vi "Get_Joystick.vi"(1 "Joystick_One":string="Pilot Controller", 2 "Joystick_Two":string="CoPilot Controller") -> (6 "Joystick_Out":T1)   [LabVIEW 2020]
uses:
  Joystick_Controls.ctl
  <vilib>/Rock Robotics/WPI/Joystick/WPI_JoystickDeviceEnum.ctl
  <vilib>/Rock Robotics/WPI/Utilities/WPI_GetSetVariantRefNum.vi
panel:
  in  "Joystick Controls":T1
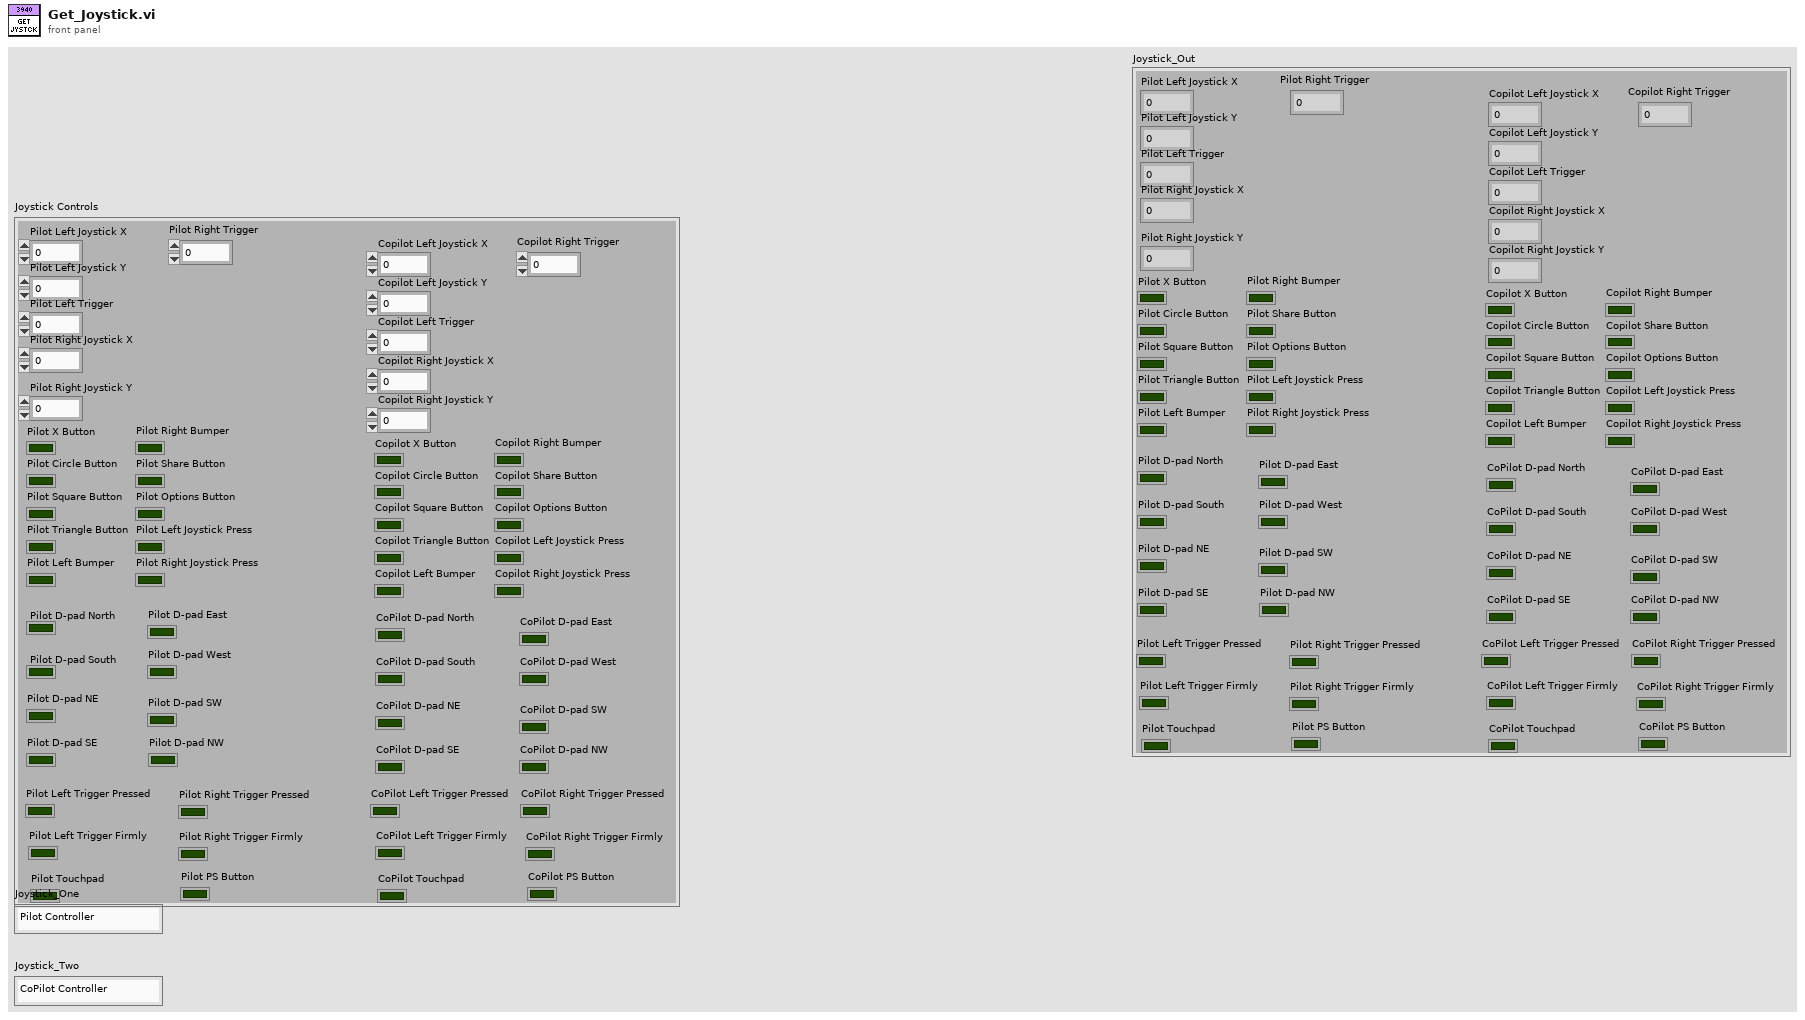
[diagram p1: front panel]
types:
  T1 = typedef "Joystick_Controls.ctl" = cluster{"Pilot Left Joystick X":dbl, "Pilot Left Joystick Y":dbl, "Pilot X Button":bool, "Pilot Circle Button":bool, "Pilot Square Button":bool, "Pilot Triangle Button":bool, "Pilot Left Bumper":bool, "Pilot Right Bumper":bool, "Pilot Share Button":bool, "Pilot Options Button":bool, "Pilot Left Joystick Press":bool, "Pilot Right Joystick Press":bool, "Pilot Left Trigger":dbl, "Pilot Right Joystick X":dbl, "Pilot Right Joystick Y":dbl, "Pilot Right Trigger":dbl, "Copilot Left Joystick X":dbl, "Copilot Left Joystick Y":dbl, "Copilot X Button":bool, "Copilot Circle Button":bool, "Copilot Square Button":bool, "Copilot Triangle Button":bool, "Copilot Left Bumper":bool, "Copilot Right Bumper":bool, "Copilot Share Button":bool, "Copilot Options Button":bool, "Copilot Left Joystick Press":bool, "Copilot Right Joystick Press":bool, "Copilot Left Trigger":dbl, "Copilot Right Joystick X":dbl, "Copilot Right Joystick Y":dbl, "Copilot Right Trigger":dbl, "Pilot D-pad North":bool, "Pilot D-pad South":bool, "Pilot D-pad East":bool, "Pilot D-pad West":bool, "Pilot D-pad NE ":bool, "Pilot D-pad SE":bool, "Pilot D-pad SW":bool, "Pilot D-pad NW":bool, "CoPilot D-pad North":bool, "CoPilot D-pad South":bool, "CoPilot D-pad East":bool, "CoPilot D-pad West":bool, "CoPilot D-pad NE":bool, "CoPilot D-pad SE":bool, "CoPilot D-pad SW":bool, "CoPilot D-pad NW":bool, "Pilot Left Trigger Pressed":bool, "Pilot Right Trigger Pressed":bool, "CoPilot Left Trigger Pressed":bool, "CoPilot Right Trigger Pressed":bool, "Pilot Left Trigger Firmly":bool, "Pilot Right Trigger Firmly":bool, "Pilot Touchpad":bool, "Pilot PS Button":bool, "CoPilot Left Trigger Firmly":bool, "CoPilot Right Trigger Firmly":bool, "CoPilot Touchpad":bool, "CoPilot PS Button":bool}
  T2 = typedef "WPI_JoystickDeviceEnum.ctl" = enum16{"USB 0", "USB 1", "USB 2", "USB 3", "USB 4", "USB 5"}
  T3 = typedef "WPI_Joystick Info.ctl" = cluster{"Device Name":string, "HID Type":T4, "XBox Type":T5, "Axes Count":i32, "Axes Types":T6[], "Button Count":i32, "POV Count":i32}
  T4 = typedef "WPI_JoystickHID Types.ctl" = enum16{"Not HID", "HID Joystick", "HID Gamepad", "HID Driving Wheel", "HID Flightstick", "HID First Person"}
  T5 = typedef "WPI_JoystickXBox Types.ctl" = enum16{"Not XBox", "XBox Unknown", "XBox Gamepad", "XBox Wheel", "XBox Arcade Stick", "XBox Flight Stick", "XBox Dance Pad", "XBox Guitar", "XBox Drum Kit", "XBox Arcade Pad"}
  T6 = typedef "WPI_JoystickAxis Types.ctl" = enum16{"X Axis", "Y Axis", "Z Axis", "RxAxis", "RyAxis", "RzAxis", "Slider", "POV", "None", "L X Axis", "L Y Axis", "L Trigger", "R Trigger", "R X Axis", "R Y Axis"}
  T7 = typedef "WPI_JoystickDevRef.ctl" = cluster{"Device":T2}
  T8 = cluster{"Axes[0]":dbl, "Axes[1]":dbl, "Axes[2]":dbl, "Axes[3]":dbl, "Axes[4]":dbl, "Axes[5]":dbl, "Axes[6]":dbl, "Axes[7]":dbl, "Axes[8]":dbl}
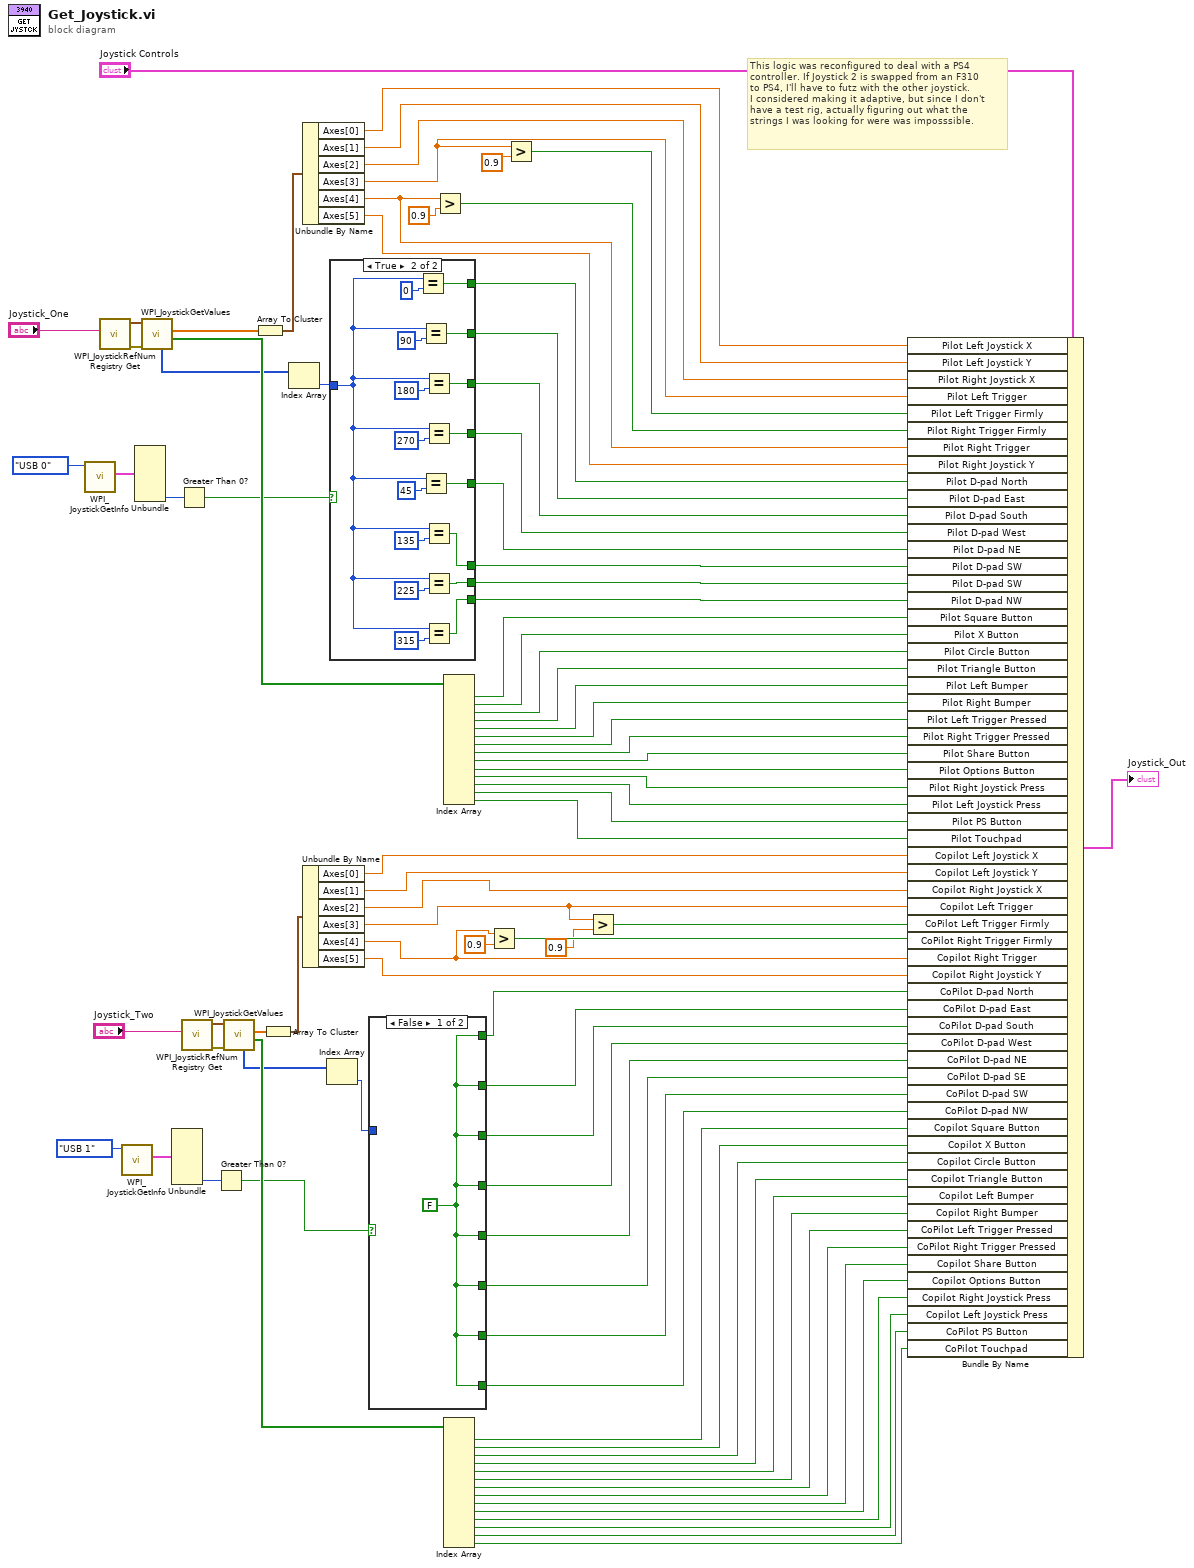
[diagram p0: block diagram]
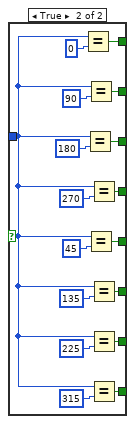
[diagram p2: hidden frame]
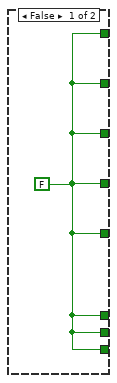
[diagram p3: hidden frame]
diagram:
  # "This logic was reconfigured to deal with a PS4\ncontroller. If Joystick 2 is swapped from an F310\nto PS4, I'll have to futz with the other joystick.\nI considered making it adaptive, but since I don't\nhave a test rig, actually figuring out what the\nstrings I was looking for were was imposssible."
  n1 = call <vilib>:"WPI_JoystickGetInfo.vi"("JoystickDevice"=WPI_JoystickDeviceEnum."USB 0") -> ("Joystick Info"=w31:T3)  [unwired: 9 in, 1 out]
  n2 = call <vilib>:"WPI_JoystickRefNum Registry Get.vi"("refnum name"="Joystick_One") -> ("error out"=w56:errorcluster, "JoystickDevRef"=w90:T7)  [unwired: 9 in]
  n3 = call <vilib>:"WPI_JoystickGetInfo.vi"("JoystickDevice"=WPI_JoystickDeviceEnum."USB 1") -> ("Joystick Info"=w27:T3)  [unwired: 9 in, 1 out]
  n4 = Unbundle(w31) -> ("POV Count"=w30:i32)  [unwired: 6 out]
  n5 = call <vilib>:"WPI_JoystickGetValues.vi"("error in (no error)"=w56, "JoystickDevRef"=w90) -> ("Buttons"=w85:bool[], "Axes"=w89:dbl[], "POVs"=w58:i16[])  [unwired: 5 in, 2 out]
  n6 = Unbundle(w27) -> ("POV Count"=w26:i32)  [unwired: 6 out]
  n7 = Greater Than 0?(x=w30) -> (x > 0?=w29:bool)
  n8 = call <vilib>:"WPI_JoystickRefNum Registry Get.vi"("refnum name"="Joystick_Two") -> ("error out"=w55:errorcluster, "JoystickDevRef"=w74:T7)  [unwired: 9 in]
  n9 = Greater Than 0?(x=w26) -> (x > 0?=w25:bool)
  n10 = call <vilib>:"WPI_JoystickGetValues.vi"("error in (no error)"=w55, "JoystickDevRef"=w74) -> ("Buttons"=w72:bool[], "Axes"=w73:dbl[], "POVs"=w57:i16[])  [unwired: 5 in, 2 out]
  n11 = Array To Cluster(array=w89) -> (cluster=w88:T8)
  n12 = Array To Cluster(array=w73) -> (cluster=w71:T8)
  n13 = Index Array(array=w58) -> (element=w45:i16)  [unwired: 1 in]
  n14 = Unbundle By Name(w88) -> ("Axes[0]"=w87:dbl, "Axes[1]"=w11:dbl, "Axes[2]"=w24:dbl, "Axes[3]"=w23:dbl, "Axes[4]"=w21:dbl, "Axes[5]"=w86:dbl)
  n15 = Unbundle By Name(w71) -> ("Axes[0]"=w18:dbl, "Axes[1]"=w17:dbl, "Axes[2]"=w35:dbl, "Axes[3]"=w6:dbl, "Axes[4]"=w9:dbl, "Axes[5]"=w70:dbl)
  n16 = Index Array(array=w57) -> (element=w37:i16)  [unwired: 1 in]
  n17 = case shown="True" w29 {
    tunnel: [w91 w108] -> w52
    tunnel: [w91 w107] -> w51
    tunnel: [w91 w106] -> w50
    tunnel: [w91 w105] -> w49
    tunnel: [w91 w104] -> w48
    tunnel: [w91 w103] -> w47
    tunnel: [w91 w102] -> w46
    tunnel: w45 -> [_ w92]
    tunnel: [w91 w93] -> w33
    frame False {
      w91 = FALSE
    }
    frame True {
      n18 = Equal?(x=w92, y=i16 0) -> (x = y?=w93:bool)
      n19 = Equal?(x=w92, y=i16 90) -> (x = y?=w108:bool)
      n20 = Equal?(x=w92, y=i16 45) -> (x = y?=w104:bool)
      n21 = Equal?(x=w92, y=i16 180) -> (x = y?=w107:bool)
      n22 = Equal?(x=w92, y=i16 270) -> (x = y?=w106:bool)
      n23 = Equal?(x=w92, y=i16 135) -> (x = y?=w103:bool)
      n24 = Equal?(x=w92, y=i16 225) -> (x = y?=w102:bool)
      n25 = Equal?(x=w92, y=i16 315) -> (x = y?=w105:bool)
    }
  }
  n26 = case shown="False" w25 {
    tunnel: [w109 w118] -> w16
    tunnel: [w109 w117] -> w44
    tunnel: [w109 w110] -> w43
    tunnel: [w109 w116] -> w42
    tunnel: [w109 w115] -> w41
    tunnel: [w109 w114] -> w40
    tunnel: [w109 w113] -> w39
    tunnel: [w109 w112] -> w38
    tunnel: w37 -> [_ w111]
    frame False {
      w109 = FALSE
    }
    frame True {
      n27 = Equal?(x=w111, y=i16 0) -> (x = y?=w118:bool)
      n28 = Equal?(x=w111, y=i16 180) -> (x = y?=w110:bool)
      n29 = Equal?(x=w111, y=i16 90) -> (x = y?=w117:bool)
      n30 = Equal?(x=w111, y=i16 45) -> (x = y?=w115:bool)
      n31 = Equal?(x=w111, y=i16 270) -> (x = y?=w116:bool)
      n32 = Equal?(x=w111, y=i16 135) -> (x = y?=w114:bool)
      n33 = Equal?(x=w111, y=i16 225) -> (x = y?=w113:bool)
      n34 = Equal?(x=w111, y=i16 315) -> (x = y?=w112:bool)
    }
  }
  n35 = Greater?(x=w21, y=0.9) -> (0:w19:bool)
  n36 = Index Array(array=w85) -> (element #1=w84:bool, element #2=w83:bool, element #3=w82:bool, element #4=w81:bool, element #5=w80:bool, element #6=w79:bool, element #7=w78:bool, element #8=w77:bool, element #9=w76:bool, element #10=w75:bool, element #11=w15:bool, element #12=w14:bool, element #13=w13:bool, element #14=w12:bool)  [unwired: 14 in]
  n37 = Index Array(array=w72) -> (element #1=w69:bool, element #2=w68:bool, element #3=w67:bool, element #4=w66:bool, element #5=w64:bool, element #6=w65:bool, element #7=w63:bool, element #8=w62:bool, element #9=w61:bool, element #10=w60:bool, element #11=w4:bool, element #12=w3:bool, element #13=w2:bool, element #14=w1:bool)  [unwired: 14 in]
  n38 = Greater?(x=w9, y=0.9) -> (0:w8:bool)
  n39 = Greater?(x=w23, y=0.9) -> (0:w22:bool)
  n40 = Greater?(x=w6, y=0.9) -> (0:w5:bool)
  n41 = Bundle By Name(cluster="Joystick Controls", "Pilot Left Joystick X"=w87, "Pilot Left Joystick Y"=w11, "Pilot Right Joystick X"=w24, "Pilot Left Trigger"=w23, "Pilot Left Trigger Firmly"=w22, "Pilot Right Trigger Firmly"=w19, "Pilot Right Trigger"=w21, "Pilot Right Joystick Y"=w86, "Pilot D-pad North"=w33, "Pilot D-pad East"=w52, "Pilot D-pad South"=w51, "Pilot D-pad West"=w50, "Pilot D-pad NE"=w48, "Pilot D-pad SW"=w47, "Pilot D-pad SW"=w46, "Pilot D-pad NW"=w49, "Pilot Square Button"=w84, "Pilot X Button"=w83, "Pilot Circle Button"=w82, "Pilot Triangle Button"=w81, "Pilot Left Bumper"=w80, "Pilot Right Bumper"=w79, "Pilot Left Trigger Pressed"=w78, "Pilot Right Trigger Pressed"=w77, "Pilot Share Button"=w76, "Pilot Options Button"=w75, "Pilot Right Joystick Press"=w15, "Pilot Left Joystick Press"=w14, "Pilot PS Button"=w13, "Pilot Touchpad"=w12, "Copilot Left Joystick X"=w18, "Copilot Left Joystick Y"=w17, "Copilot Right Joystick X"=w35, "Copilot Left Trigger"=w6, "CoPilot Left Trigger Firmly"=w5, "CoPilot Right Trigger Firmly"=w8, "Copilot Right Trigger"=w9, "Copilot Right Joystick Y"=w70, "CoPilot D-pad North"=w16, "CoPilot D-pad East"=w44, "CoPilot D-pad South"=w43, "CoPilot D-pad West"=w42, "CoPilot D-pad NE"=w41, "CoPilot D-pad SE"=w40, "CoPilot D-pad SW"=w39, "CoPilot D-pad NW"=w38, "Copilot Square Button"=w69, "Copilot X Button"=w68, "Copilot Circle Button"=w67, "Copilot Triangle Button"=w66, "Copilot Left Bumper"=w64, "Copilot Right Bumper"=w65, "CoPilot Left Trigger Pressed"=w63, "CoPilot Right Trigger Pressed"=w62, "Copilot Share Button"=w61, "Copilot Options Button"=w60, "Copilot Right Joystick Press"=w4, "Copilot Left Joystick Press"=w3, "CoPilot PS Button"=w2, "CoPilot Touchpad"=w1) -> (→"Joystick_Out":T1)
